vi "Append tiff file with existing Tiff file or Tiff string.vi"(0 "Existing Tiff File (A) refnum":refnum<file>, 1 "IsTIFF?\n(Check file)":bool, 2 "Litt/BigEnd":bool, 5 "Tiff file (B)":path, 7 "Tiff file (B)\n (unsigned byte array)":u8[](array[numeric]), 9 "Location in existing file of\nit's last page's \n\"next IFD pointer\"":i64, 11 "error in":errorcluster) -> (4 "File refnum out":refnum<file>, 10 "Location in new file of\nit's last page's \n\"next IFD pointer\"":i64, 15 "error out":errorcluster)   [LabVIEW 2015, in "Tiff reader.lvlib"]
doc: "This .vi appends a single TIF image (B) into an exisitng TIF file (A) (which can be an image or a stack). The TIFF image (B) to append can be either a string or an existing file on disk.\n\nThe location of the TIF file (A)'s \"next IFD pointer\" must be input into this VI. That is obtained by either using the \"Find last IFD.vi\" or by using the output of this VI (if you are sequentially appending multiple images in a row)."
uses:
  Tiff reader.lvlib
panel:
  out "existing file size(s)":i64
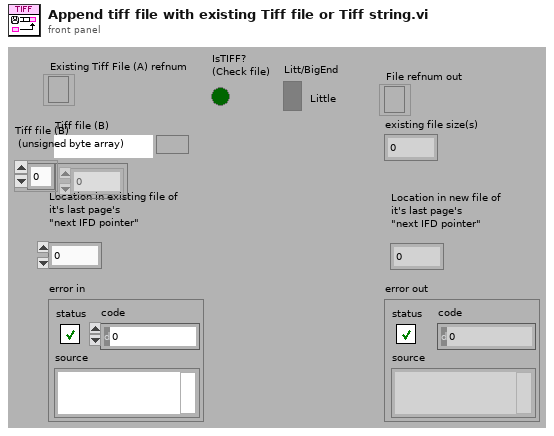
[diagram p1: front panel]
types:
  T1 = typedef "Tiff reader.lvlib/IFD Entry.ctl" = cluster{"Tag":u16, "Type":T2, "Count":u32, "Val/Offs":u32, "Is Pointer?":bool, "Byte stream index":i32}
  T2 = typedef "Tiff reader.lvlib/FieldTypes.ctl" = enum16{"NULL", "U8", "ASCII7", "U16", "U32", "RATIONAL", "SByte(I8)", "Undef(8Bit)", "I16", "I32", "SRat(4B:4B)", "SGL(4Byte)", "DBL(8Byte)"}
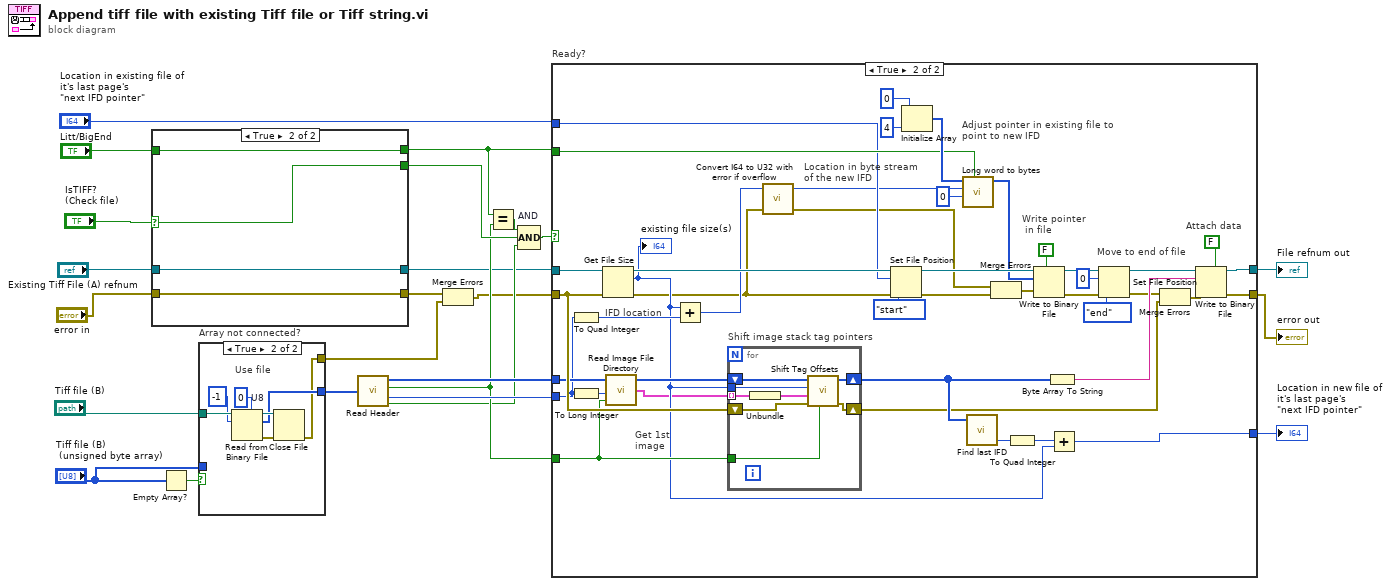
[diagram p0: block diagram]
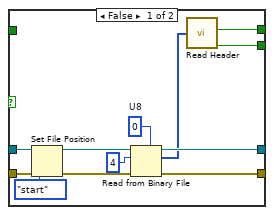
[diagram p2: hidden frame]
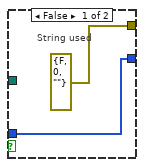
[diagram p3: hidden frame]
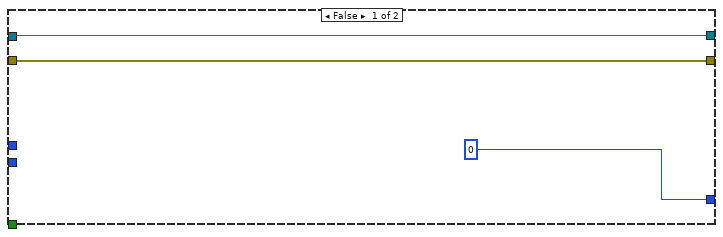
[diagram p4: hidden frame]
diagram:
  n1 = case shown="True" "IsTIFF?\n(Check file)" {
    selector: "IsTIFF?\n(Check file)" -> [_ w38]
    tunnel: [w36 w38] -> w22
    tunnel: [w35 w37] -> w20
    tunnel: "Existing Tiff File (A) refnum" -> [w31 w39]
    tunnel: "error in" -> [w30 w40]
    tunnel: [w29 w39] -> w11
    tunnel: [w25 w40] -> w5
    tunnel: "Litt/BigEnd" -> [_ w37]
    frame False {
      w27 = u8 0  # U8
      n2 = Set File Position(refnum=w31, from (0:start)=enum16{"start", "end", "current"}."start", error in=w30) -> (refnum out=w32:refnum<file>, error out=w28:errorcluster)  [unwired: 1 in]
      n3 = Read from Binary File(5:w27, 8:w28, 10:4 ("count (1)"), 11:w32) -> (0:w25:errorcluster, 2:w26:u8[], 3:w29:refnum<file>)  [unwired: 3 out]
      n4 = call "Read Header.vi"("TIFF Data in"=w26) -> ("Litt/BigEnd"=w35:bool, "IsTIFF?"=w36:bool)  [unwired: 2 out]
    }
    frame True {
    }
  }
  n5 = Empty Array?(array="Tiff file (B)\n (unsigned byte array)") -> (empty?=w9:bool)
  n6 = case "Array not connected?" shown="True" w9 {
    tunnel: "Tiff file (B)" -> [_ w49]
    tunnel: [w41 w46] -> w6
    tunnel: "Tiff file (B)\n (unsigned byte array)" -> [w41 _]
    tunnel: [errorcluster {"status"=FALSE, "code"=0, "source"=""} ("error out") w44] -> w4
    frame False {
      # "String used"
    }
    frame True {
      w43 = u8 0  # U8
      # "Use file"
      n7 = Read from Binary File(5:w43, 10:-1 ("count (1)"), 11:w49) -> (0:w48:errorcluster, 2:w46:u8[], 3:w47:refnum<file>)  [unwired: 1 in, 3 out]
      n8 = Close File(refnum=w47, error in=w48) -> (error out=w44:errorcluster)  [unwired: 1 out]
    }
  }
  n9 = call "Read Header.vi"("TIFF Data in"=w6) -> ("TIFF Data out"=w23:u8[], "Litt/BigEnd"=w19:bool, "ImFileDirectOffs"=w24:u32, "IsTIFF?"=w18:bool)
  n10 = Merge Errors(w5, w4) -> (w3:errorcluster)
  n11 = Equal?(x=w20, y=w19) -> (x = y?=w21:bool)
  n12 = Compound Arithmetic op=AND "AND"(w21, w22, w18) -> (w17:bool)
  n13 = case "Ready?" shown="True" w17 {
    tunnel: w24 -> [_ w53]
    tunnel: w23 -> [_ w94]
    tunnel: w20 -> [_ w85]
    tunnel: w19 -> [_ w71]
    tunnel: [u32 0 w75] -> w16
    tunnel: [w51 w74] -> w14
    tunnel: w11 -> [w52 w73]
    tunnel: [w52 w72] -> w15
    tunnel: w3 -> [w51 w95]
    tunnel: "Location in existing file of\nit's last page's \n\"next IFD pointer\"" -> [_ w69]
    frame False {
    }
    frame True {
      # "IFD location"
      # "Move to end of file"
      # "Write pointer\n in file"
      # "Attach data"
      # "Adjust pointer in existing file to\npoint to new IFD"
      # "Location in byte stream\nof the new IFD"
      # "Get 1st\nimage"
      n14 = To Quad Integer(1:w53) -> (0:w68:i64)
      n15 = To Long Integer(number=w53) -> (32bit integer=w54:i32)
      n16 = Get File Size(file=w73, error in=w95) -> (refnum out=w89:refnum<file>, size (in bytes)=w63:i64, 0:w61:errorcluster)
      "existing file size(s)" <- w63
      n17 = call "Read Image File Directory.vi"("Litt/BigEnd"=w71, "Im_File_Dir Offs"=w54, "Image Data in"=w94) -> ("Directories"=w62:cluster{"Tags":T1[]}[], "Image Data out"=w93:u8[])  [unwired: 1 out]
      n18 = Add(x=w63, y=w68) -> (x+y=w67:i64)
      n19 = for "Shift image stack tag pointers" {
        tunnel: w71 -> [w101]
        tunnel: w63 -> [w98]
        shift-right: [w100] -> w70
        shift-left: w93 -> [w102]
        shift-right: [w99] -> w60
        shift-left: w95 -> [w103]
        tunnel: w62 -> [w97] mode=indexing
        n20 = Unbundle(w97) -> ("Tags"=w96:T1[])
        n21 = call "Shift Tag Offsets.vi"("Litt/BigEnd"=w101, "error in"=w103, "Tags"=w96, "# of bytes inserted before tag data"=w98, "Image Data"=w102) -> ("error out"=w99:errorcluster, "Image Data Out"=w100:u8[])  [unwired: 4 in, 1 out]
      }
      n22 = call "Convert I64 to U32 with error if overflow.vi"("error in"=w61, "I64"=w67) -> ("error out"=w57:errorcluster, "U32"=w66:u32)  [unwired: 2 out]
      n23 = Set File Position(offset (in bytes) (0)=w69, refnum=w89, from (0:start)=enum16{"start", "end", "current"}."start", error in=w61) -> (refnum out=w88:refnum<file>, error out=w56:errorcluster)
      n24 = Initialize Array(u8 0 ("dimension size"), 4 ("dimension size")) -> (w92:u8[])
      n25 = call "Long word to bytes.vi"("Litt/BigEnd"=w85, "Index"=0, "U32"=w66, "Image Data in"=w92) -> ("Image Data out"=w87:u8[])  [unwired: 5 out]
      n26 = call "Find last IFD.vi"("TIFF Data in"=w70) -> ("Location in byte stream of last IFD pointer.  This\nis the word to change if you are adding another page\nto the file."=w65:i32)  [unwired: 4 out]
      n27 = Merge Errors(w57, w56) -> (w55:errorcluster)
      n28 = To Quad Integer(1:w65) -> (0:w64:i64)
      n29 = Write to Binary File(file (use dialog)=w88, data=w87, error in=w55, 5:FALSE ("prepend array or string size? (T)")) -> (refnum out=w83:refnum<file>, error out=w84:errorcluster)  [unwired: 3 out]
      n30 = Byte Array To String(unsigned byte array=w70) -> (string=w78:string)
      n31 = Add(x=w64, y=w63) -> (x+y=w75:i64)
      n32 = Set File Position(offset (in bytes) (0)=i64 0, refnum=w83, from (0:start)=enum16{"start", "end", "current"}."end", error in=w84) -> (refnum out=w79:refnum<file>, error out=w59:errorcluster)
      n33 = Merge Errors(w59, w60) -> (w58:errorcluster)
      n34 = Write to Binary File(file (use dialog)=w79, data=w78, error in=w58, 5:FALSE ("prepend array or string size? (T)")) -> (refnum out=w72:refnum<file>, error out=w74:errorcluster)  [unwired: 3 out]
    }
  }
  "Location in new file of\nit's last page's \n\"next IFD pointer\"" <- w16
  "File refnum out" <- w15
  "error out" <- w14
